vi "XY Graph Interpolate Plot at x.vi"(8 "Error In":errorcluster, 9 "XY Plot":T1, 11 "t":dbl format="%#_4g") -> (0 "Error Out":errorcluster, 3 "XY Plot(t)":dbl format="%#_4g")   [LabVIEW 2021, in "XY Graph Add-Ons.lvlib"]
doc: "Compute the value G(t) where t is the input time point and User-defined Gate is a cluster of two arrays, [t_i], i = 0, ..., n and [G_i}, i = 0,..., n as:\n1) G(t) = 0 if t < t_0 or t > t_n\n2) G(t) is linearly interpolated in between"
uses:
  XY Graph Add-Ons.lvlib
  XY Graph Plot Data.ctl
  <vilib>/Utility/error.llb/Error Cluster From Error Code.vi
  <vilib>/ErrorRing/Error Ring.xnode
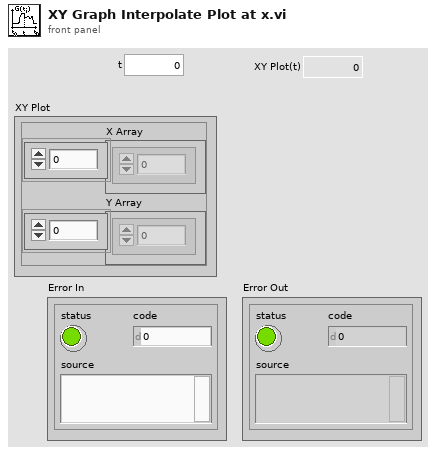
[diagram p1: front panel]
types:
  T1 = typedef "XY Graph Add-Ons.lvlib/XY Graph Plot Data.ctl" = cluster{"X Array":dbl[], "Y Array":dbl[]}
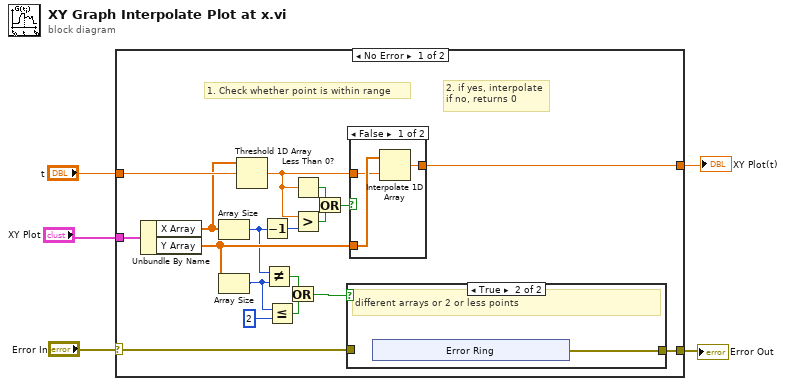
[diagram p0: block diagram]
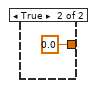
[diagram p3: hidden frame]
diagram:
  n1 = case shown="No Error" "Error In" {
    selector: "Error In" -> [w8 w34]
    tunnel: "t" -> [w23 _]
    tunnel: [w22 _] -> w4
    tunnel: "XY Plot" -> [w15 _]
    tunnel: [w6 w34] -> w1
    frame No Error {
      # "2. if yes, interpolate\nif no, returns 0"
      # "1. Check whether point is within range"
      n2 = Unbundle By Name(w15) -> ("X Array"=w21:dbl[], "Y Array"=w14:dbl[])
      n3 = Array Size(array=w21) -> (size(s)=w13:i32)
      n4 = Array Size(array=w14) -> (size(s)=w12:i32)
      n5 = Threshold 1D Array(2:w23, 3:w21) -> (0:w20:dbl)  [unwired: 1 in]
      n6 = Decrement(x=w13) -> (x-1=w16:i32)
      n7 = Not Equal?(x=w13, y=w12) -> (x != y?=w10:bool)
      n8 = Less Or Equal?(x=w12, y=2) -> (x <= y?=w9:bool)
      n9 = Or(x=w10, y=w9) -> (x .or. y?=w7:bool)
      n10 = Less Than 0?(x=w20) -> (x < 0?=w19:bool)
      n11 = Greater?(x=w20, y=w16) -> (0:w18:bool)
      n12 = Or(x=w19, y=w18) -> (x .or. y?=w17:bool)
      n13 = case shown="True" w7 {
        tunnel: w8 -> [w24 _]
        tunnel: [w24 w25] -> w6
        frame False {
        }
        frame True {
          # "different arrays or 2 or less points"
          n14 = xnode "Error Ring"() -> ("error out"=w25:errorcluster)
        }
      }
      n15 = case shown="False" w17 {
        tunnel: w14 -> [w32 _]
        tunnel: [w31 0.0] -> w22
        tunnel: w20 -> [w30 _]
        frame False {
          n16 = Interpolate 1D Array(1:w30, 2:w32) -> (0:w31:dbl)
        }
        frame True {
        }
      }
    }
    frame Error {
    }
  }
  "XY Plot(t)" <- w4
  "Error Out" <- w1
